vi "模式树更新.vi"(8 "错误输入（无错误）":errorcluster, 10 "模式列表-new":T1(array[cluster]) {"sce-pannel-list"."pannel"."ID" format="%02x"}, 11 "模式树形引用":refnum<vi>) -> (0 "错误输出":errorcluster, 3 "引用输出":refnum<vi>)   [LabVIEW 2019]
panel:
  out "编辑树形控件项:添加项":string
  in  "场景":string(tree)
  in  "模式":string(tree)
  in  "模式列表":T2(array[cluster])
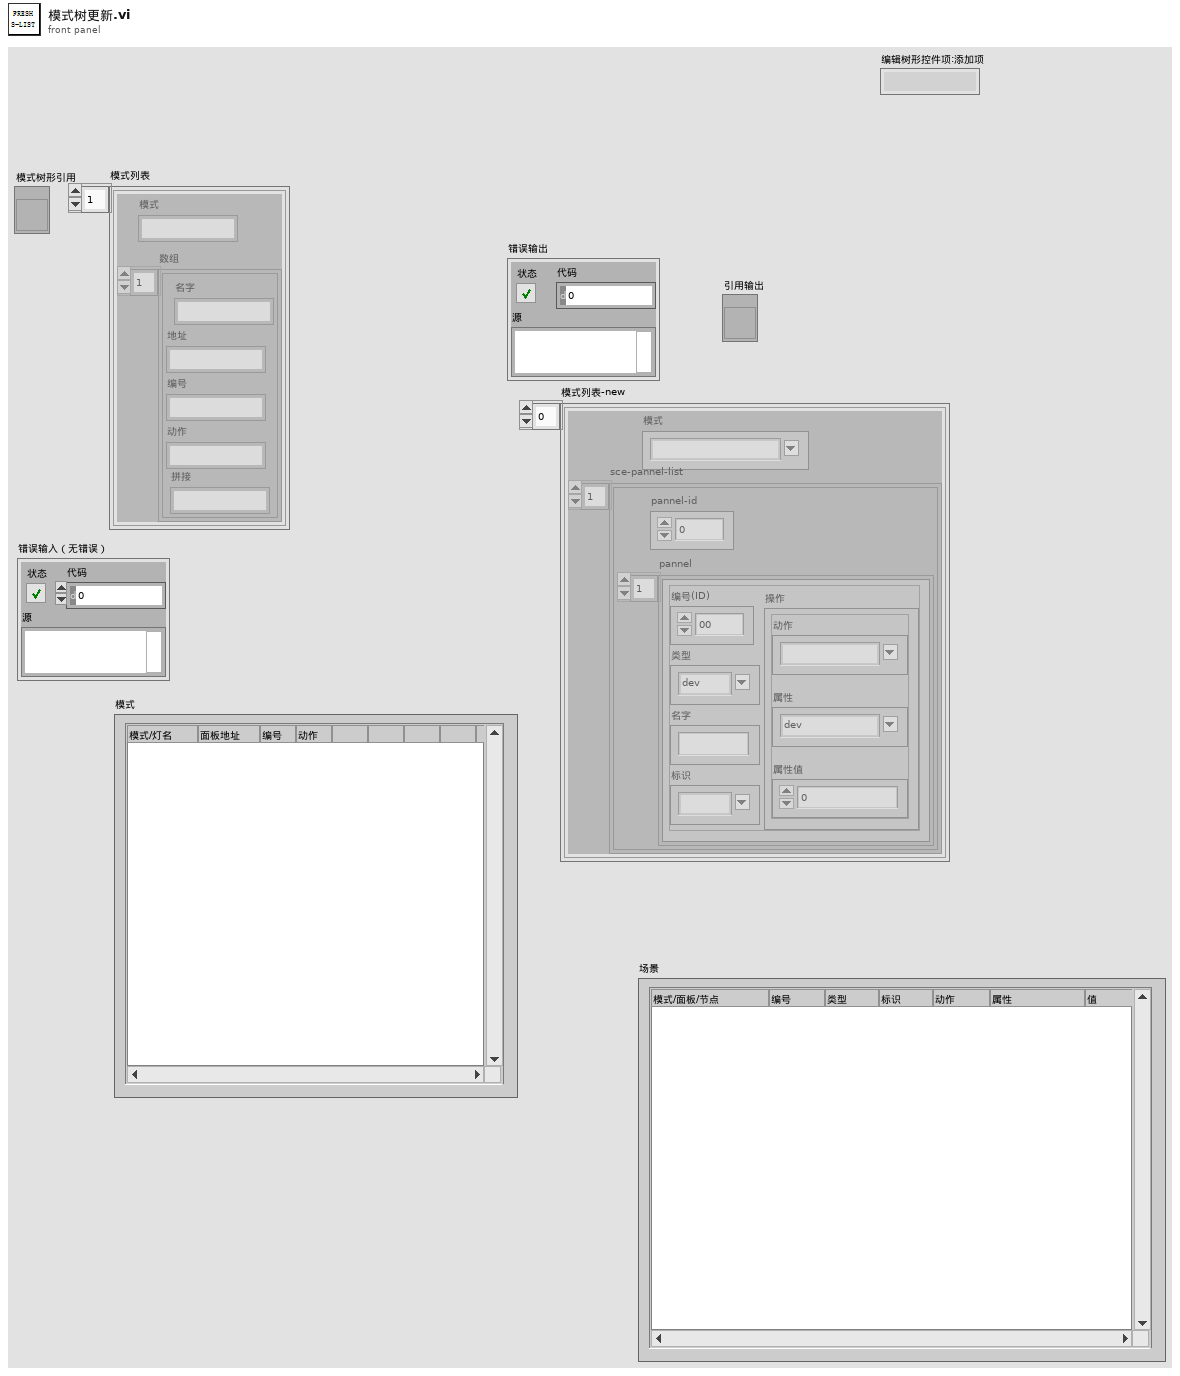
[diagram p1: front panel]
types:
  T1 = cluster{"模式":string, "sce-pannel-list":cluster{"pannel":cluster{"ID":u8, "type":string, "flag":string, "name":string, "Act":cluster{"Attribute":string, "Action":string, "Value":dbl}}[], "pannel-id":dbl}[]}[]
  T2 = cluster{"模式":string, "数组":cluster{"地址":string, "名字":string, "编号":string, "动作":string, "拼接":string}[]}[]
  T3 = cluster{"地址":string, "名字":string, "编号":string, "动作":string, "拼接":string}[]
  T4 = cluster{"pannel":cluster{"ID":u8, "type":string, "flag":string, "name":string, "Act":cluster{"Attribute":string, "Action":string, "Value":dbl}}[], "pannel-id":dbl}[]
  T5 = cluster{"ID":u8, "type":string, "flag":string, "name":string, "Act":cluster{"Attribute":string, "Action":string, "Value":dbl}}[]
  T6 = cluster{"Attribute":string, "Action":string, "Value":dbl}
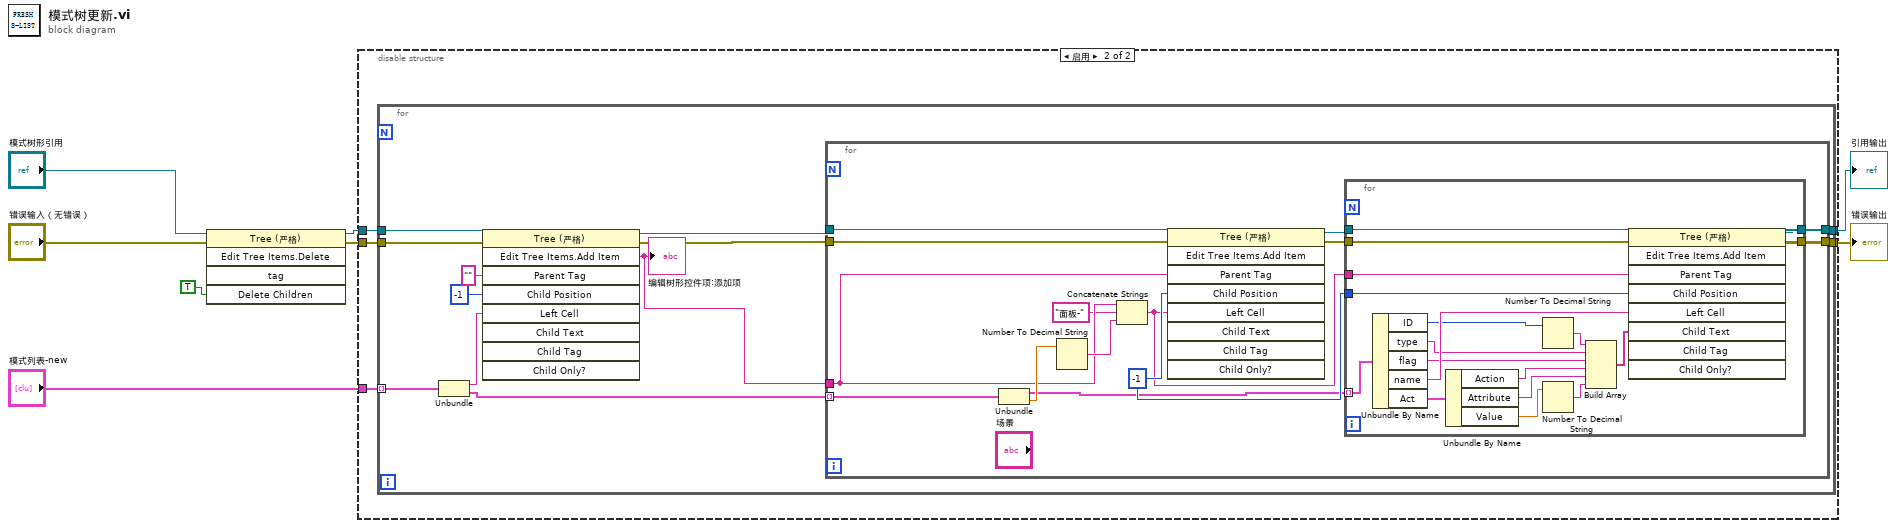
[diagram p0: block diagram]
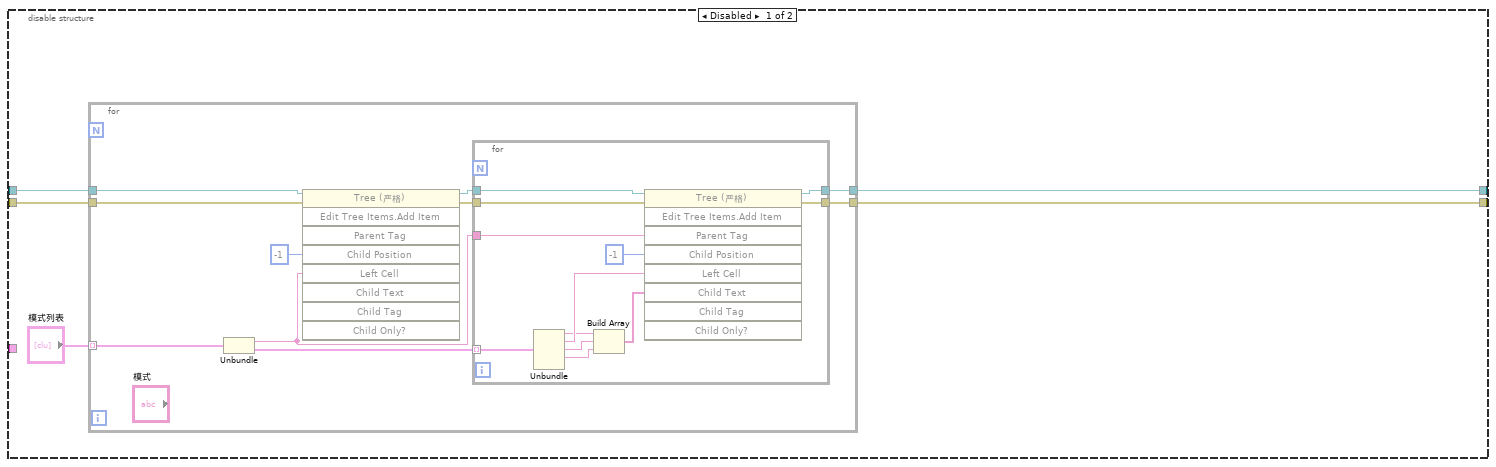
[diagram p2: hidden frame]
diagram:
  n1 = invoke class="Tree (严格)" method="Edit Tree Items.Delete"(reference="模式树形引用", error in="错误输入（无错误）", "Delete Children"=TRUE ("删除子项？")) -> (reference out=w7:refnum<vi>, error out=w4:errorcluster)  [unwired: 2 in, 3 out]
  n2 = disable-structure shown="启用" {
    disable-tunnel: w7 -> [w13 w40]
    disable-tunnel: w4 -> [w11 w36]
    disable-tunnel: [w10 w38] -> w1
    disable-tunnel: [w9 w37] -> w3
    disable-tunnel: "模式列表-new" -> [_ w39]
    frame Disabled {
      n3 = for {
        tunnel: w13 -> [w22]
        tunnel: "模式列表" -> [w21] mode=indexing
        tunnel: w11 -> [w18]
        tunnel: [w16] -> w10
        tunnel: [w15] -> w9
        n4 = Unbundle(w21) -> ("模式"=w14:string, "数组"=w20:T3)
        n5 = invoke class="Tree (严格)" method="Edit Tree Items.Add Item"(reference=w22, error in=w18, "Child Position"=-1 ("子项位置"), "Left Cell"=w14) -> (reference out=w19:refnum<vi>, error out=w17:errorcluster)  [unwired: 5 in, 7 out]
        n6 = for {
          tunnel: w20 -> [w32] mode=indexing
          tunnel: w19 -> [w34]
          tunnel: w17 -> [w33]
          tunnel: [w26] -> w16
          tunnel: [w25] -> w15
          tunnel: w14 -> [w24]
          n7 = Unbundle(w32) -> ("地址"=w30:string, "名字"=w31:string, "编号"=w29:string, "动作"=w28:string)  [unwired: 1 out]
          n8 = Build Array(w30, w29, w28) -> (w27:string[])
          n9 = invoke class="Tree (严格)" method="Edit Tree Items.Add Item"(reference=w34, error in=w33, "Parent Tag"=w24, "Child Position"=-1 ("子项位置"), "Left Cell"=w31, "Child Text"=w27) -> (reference out=w26:refnum<vi>, error out=w25:errorcluster)  [unwired: 3 in, 7 out]
        }
      }
    }
    frame Enabled {
      n10 = for {
        tunnel: w40 -> [w51]
        tunnel: w39 -> [w50] mode=indexing
        tunnel: [w46] -> w38
        tunnel: [w45] -> w37
        tunnel: w36 -> [w43]
        n11 = Unbundle(w50) -> ("模式"=w48:string, "sce-pannel-list"=w49:T4)
        n12 = invoke class="Tree (严格)" method="Edit Tree Items.Add Item"(reference=w51, error in=w43, "Parent Tag"="" ("父项标识符"), "Child Position"=-1 ("子项位置"), "Left Cell"=w48) -> (reference out=w47:refnum<vi>, error out=w44:errorcluster, "Edit Tree Items:Add Item"=w41:string)  [unwired: 4 in, 6 out]
        "编辑树形控件项:添加项" <- w41
        n13 = for {
          tunnel: w49 -> [w66] mode=indexing
          tunnel: w41 -> [w63]
          tunnel: w47 -> [w61]
          tunnel: [w56] -> w46
          tunnel: [w55] -> w45
          tunnel: w44 -> [w53]
          w59 = -1 ("子项位置")
          n14 = Unbundle(w66) -> ("pannel"=w57:T5, "pannel-id"=w65:dbl)
          n15 = Number To Decimal String(number=w65) -> (decimal integer string=w64:string)  [unwired: 1 in]
          n16 = Concatenate Strings(w63, "面板-" ("字符串"), w64) -> (w58:string)
          n17 = invoke class="Tree (严格)" method="Edit Tree Items.Add Item"(reference=w61, error in=w53, "Parent Tag"=w63, "Child Position"=w59, "Left Cell"=w58) -> (reference out=w60:refnum<vi>, error out=w54:errorcluster)  [unwired: 4 in, 7 out]
          n18 = for {
            tunnel: w60 -> [w84]
            tunnel: w59 -> [w83]
            tunnel: w58 -> [w82]
            tunnel: w57 -> [w81] mode=indexing
            tunnel: [w69] -> w56
            tunnel: [w68] -> w55
            tunnel: w54 -> [w67]
            n19 = Unbundle By Name(w81) -> ("ID"=w79:u8, "type"=w77:string, "flag"=w76:string, "name"=w80:string, "Act"=w75:T6)
            n20 = Unbundle By Name(w75) -> ("Action"=w73:string, "Attribute"=w72:string, "Value"=w74:dbl)
            n21 = Number To Decimal String(number=w79) -> (decimal integer string=w78:string)  [unwired: 1 in]
            n22 = Number To Decimal String(number=w74) -> (decimal integer string=w71:string)  [unwired: 1 in]
            n23 = Build Array(w78, w77, w76, w73, w72, w71) -> (w70:string[])
            n24 = invoke class="Tree (严格)" method="Edit Tree Items.Add Item"(reference=w84, error in=w67, "Parent Tag"=w82, "Child Position"=w83, "Left Cell"=w80, "Child Text"=w70) -> (reference out=w69:refnum<vi>, error out=w68:errorcluster)  [unwired: 3 in, 7 out]
          }
        }
      }
    }
  }
  "引用输出" <- w1
  "错误输出" <- w3
